vi "Change Room Name.vi"(8 "error in (no error)":errorcluster, 9 "New Name":string, 10 "Room GUID":string, 11 "Room-API in":refnum<class "Room-API.lvclass">) -> (0 "error out":errorcluster, 2 "updated?":bool, 3 "Room-API out":refnum<class "Room-API.lvclass">)   [LabVIEW 2020, in "Room-API.lvclass"]
uses:
  Room-API.lvclass
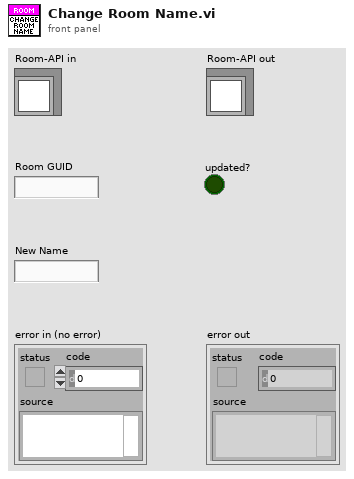
[diagram p1: front panel]
types:
  T1 = typedef "Room-API.lvclass/Single Room.ctl" = cluster{"name":string, "temperature_humidity":string[], "bond":string[], "hue":string[]}
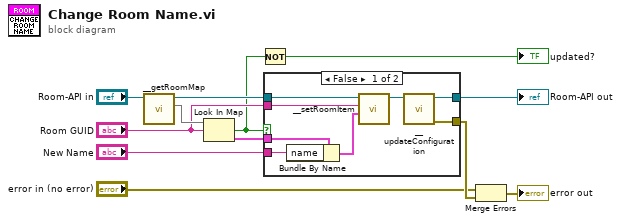
[diagram p0: block diagram]
diagram:
  n1 = call "__getRoomMap.vi"("Room-API in"="Room-API in") -> ("room_map"=w7:map{string, T1}, "Room-API out"=w10:refnum<class "Room-API.lvclass">)  [unwired: 9 in]
  n2 = Look In Map(map=w7, key="Room GUID") -> (key not found?=w5:bool, value=w11:T1)  [unwired: 1 in]
  n3 = Not(x=w5) -> (.not. x?=→"updated?":bool)
  n4 = case shown="False" w5 {
    tunnel: w11 -> [w20 _]
    tunnel: w10 -> [w18 w21]
    tunnel: [w14 w21] -> w9
    tunnel: "New Name" -> [w19 _]
    tunnel: "Room GUID" -> [w17 _]
    tunnel: [w13 _] -> w3
    frame False {
      n5 = Bundle By Name(cluster=w20, "name"=w19) -> (w16:T1)
      n6 = call "__setRoomItem.vi"("room"=w16, "Room GUID"=w17, "Room-API in"=w18) -> ("Room-API out"=w15:refnum<class "Room-API.lvclass">)  [unwired: 8 in]
      n7 = call "__updateConfiguration.vi"("Room-API in"=w15) -> ("error out"=w13:errorcluster, "Room-API out"=w14:refnum<class "Room-API.lvclass">)  [unwired: 9 in]
    }
    frame True {
    }
  }
  "Room-API out" <- w9
  n8 = Merge Errors("error in (no error)", w3) -> (→"error out":errorcluster)
